vi "generate random array.vi"() -> (3 "Random Array":dbl[](array[numeric]))   [LabVIEW 2020]
doc: "This Vi Generates a 1D array of random length with random floating numbers within given ranges."
uses:
  <vilib>/numeric/Random Number (Range) U64.vi
  <vilib>/numeric/Random Number (Range) DBL.vi
  <vilib>/numeric/sub_Random U32.vi
panel:
  in  "element upper":dbl=100.0
  in  "element lower":dbl
  out "Rand array size":i32=5
  in  "Array Size Rand Lower":u64
  in  "Array Size Rand Upper":u64=10
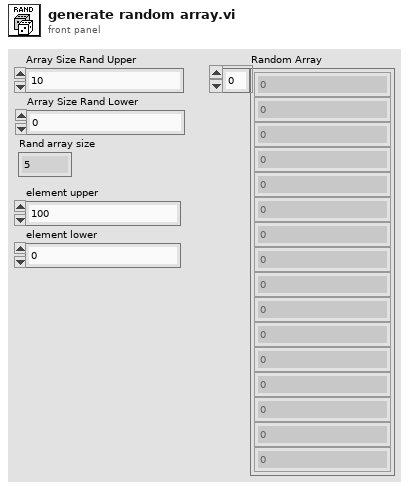
[diagram p1: front panel]
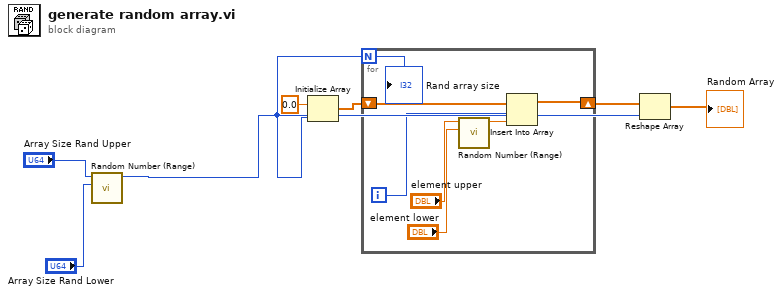
[diagram p0: block diagram]
diagram:
  n1 = call-poly <vilib>:"Random Number (Range).vi"("lower bound (0)"="Array Size Rand Lower", "upper bound (100)"="Array Size Rand Upper") -> ("number"=w2:u64)  [unwired: 9 in]
  n2 = Initialize Array(0.0 ("element"), w2) -> (w4:dbl[])
  n3 = for {
    N: w2 -> [w8]
    shift-right: [w11] -> w3
    shift-left: w4 -> [w14]
    i -> [w13]
    n4 = call-poly <vilib>:"Random Number (Range).vi"("lower bound (0)"="element lower", "upper bound (100)"="element upper") -> ("number"=w12:dbl)  [unwired: 9 in]
    n5 = Insert Into Array(array=w14, index=w13, new element=w12) -> (w11:dbl[])
    "Rand array size" <- w8
  }
  n6 = Reshape Array(w3, w2) -> (→"Random Array":dbl[])
